vi "rad7.vi"() -> ()   [LabVIEW 2012]
uses:
  <vilib>/Platform/TimedLoop/XDataNode/timing_clust.ctl
  <vilib>/Platform/TimedLoop/XDataNode/nitl_modes.ctl
  <vilib>/Platform/TimedLoop/XDataNode/wakeup.ctl
  <vilib>/Instr/_visa.llb/VISA Configure Serial Port (Instr).vi
  <vilib>/Platform/TimedLoop/XDataNode/XDataNode.xnode
  <vilib>/Platform/TimedLoop/XDataNode/XDNodeRunTimeDep.lvlib
panel:
  out "String":string
  out "Numeric 2":i32
  in  "Path":path
  in  "VISA resource name":refnum<visa-resource-name>
  in  "Command":string
  out "Numeric":i32
  in  "Loop Time (s)":dbl
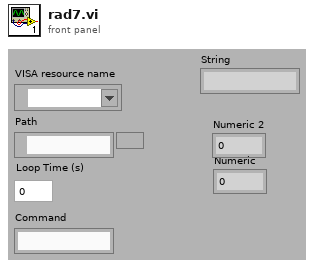
[diagram p1: front panel]
types:
  T1 = typedef "XDNodeRunTimeDep.lvlib/timing_clust.ctl" = cluster{"Expected End [f-1]":u64, "Actual End [f-1]":u64, "Finished Late? [f-1]":bool, "Expected End [i-1]":u64, "Actual End [i-1]":u64, "Finished Late? [i-1]":bool, "Expected Start [i]":u64, "Actual Start [i]":u64, "Expected Start [f]":u64, "Actual Start [f]":u64, "Source Name":string, "Structure Name":string, "Period":i64, "Deadline":i64, "Offset":i64, "Start":i64, "Priority":i32, "Timeout":i32, "Mode":T2, "Wakeup Reason":T3, "Error":errorcluster, "Source Type":string, "Secondary Source Type":string, "Global End Time":u64, "Global Start Time":u64, "Frame Duration":u64, "Iteration Duration":u64, "Assigned CPU":i32, "I/O Scan Engine Mode":u32}
  T2 = typedef "XDNodeRunTimeDep.lvlib/nitl_modes.ctl" = enum32{"No Change", "Process missed periods, maintain original phase", "Discard missed periods, maintain original phase", "Process missed periods, ignore original phase", "Discard missed periods, ignore original phase"}
  T3 = typedef "XDNodeRunTimeDep.lvlib/wakeup.ctl" = enum32{"Normal", "Aborted", "Asynchronous wakeup", "Timing source error", "Timed loop error", "Timeout"}
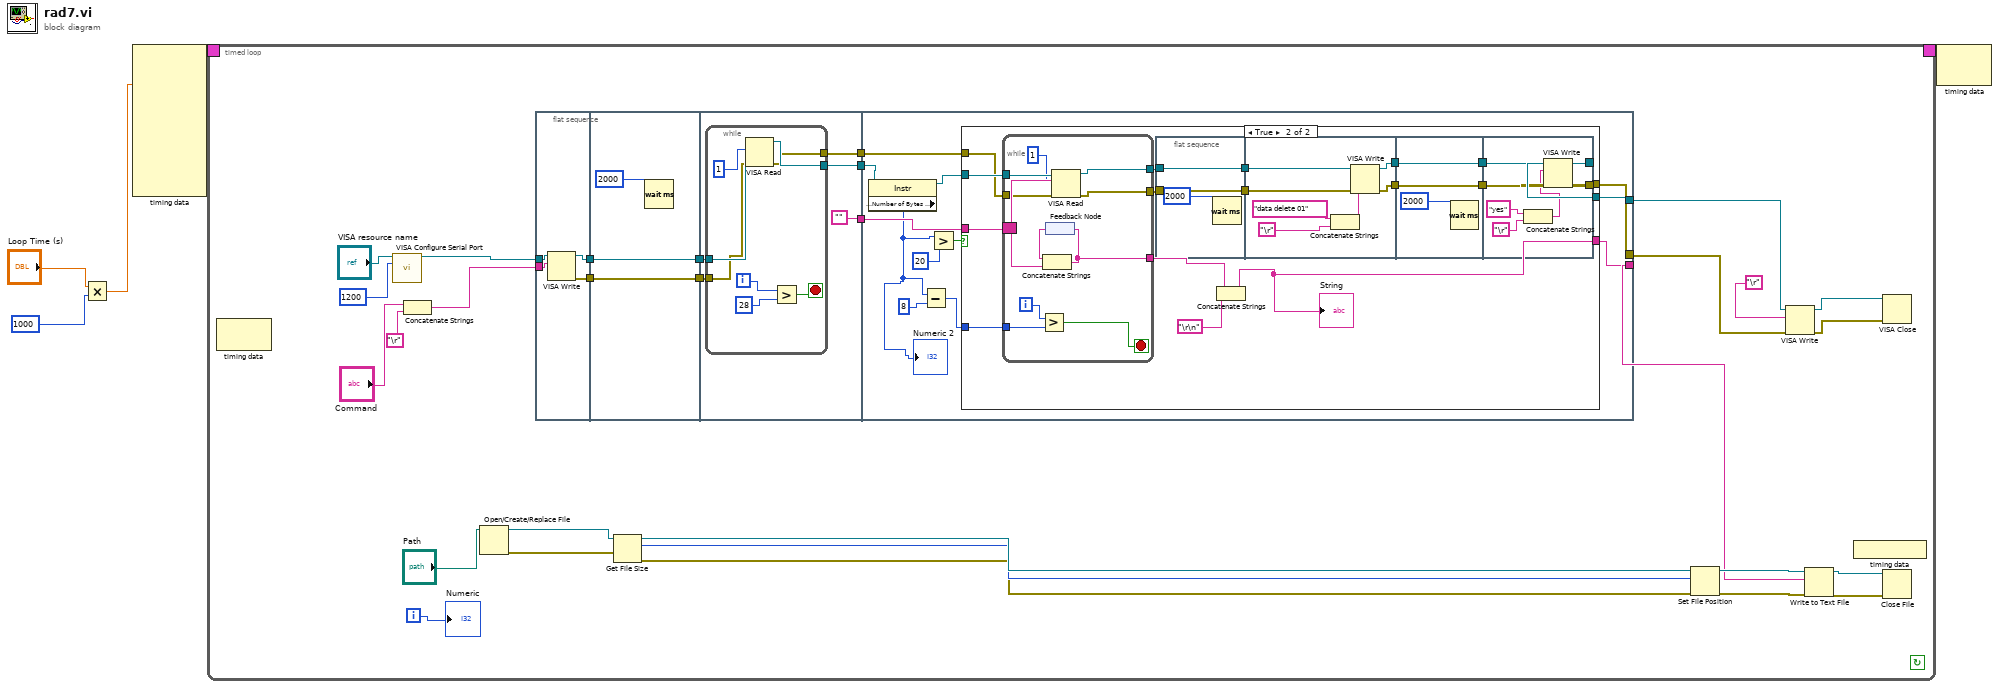
[diagram p0: block diagram]
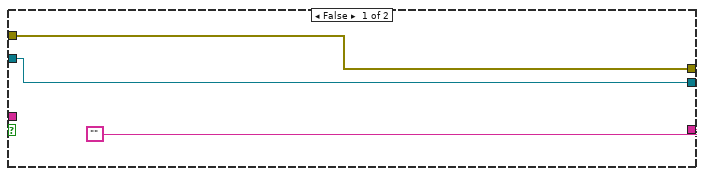
[diagram p2: hidden frame]
diagram:
  n1 = Multiply(x="Loop Time (s)", y=1000) -> (x*y=w1:dbl)
  n2 = node-c288(w1) -> (w5:T1)  [unwired: 8 in]
  n3 = timed-loop {
    timing: w5 -> [_]
    timing-out: [_] -> w4
    i -> [w30]
    stop <- _ continue-if-true
    n4 = node-c288() -> ()  [unwired: 1 in, 1 out]
    n5 = call-poly "VISA Configure Serial Port"("VISA resource name"="VISA resource name", "baud rate (9600)"=1200) -> ("VISA resource name out"=w16:refnum<visa-resource-name>)  [unwired: 12 in, 1 out]
    n6 = Concatenate Strings("Command", "\r") -> (w15:string)
    n7 = Open/Create/Replace File(file path (use dialog)="Path") -> (refnum out=w34:refnum<file>, error out=w33:errorcluster)  [unwired: 5 in, 1 out]
    n8 = flat-sequence {
      tunnel: w15 -> [w39]
      tunnel: w16 -> [w38]
      tunnel: [w37] -> w11
      tunnel: [w36] -> w9
      tunnel: w11 -> [w42]
      tunnel: [w42] -> w10
      tunnel: w9 -> [w41]
      tunnel: [w41] -> w8
      tunnel: [w47] -> w19
      tunnel: [""] -> w18
      tunnel: [w45] -> w17
      tunnel: w10 -> [w44]
      tunnel: w8 -> [w43]
      tunnel: [w67] -> w12
      tunnel: w19 -> [w65]
      tunnel: w18 -> [w66]
      tunnel: [w59] -> w13
      tunnel: w17 -> [w61]
      tunnel: [w60] -> w14
      frame #0 {
        n9 = VISA Write(VISA resource name=w38, write buffer=w39) -> (VISA resource name out=w37:refnum<visa-resource-name>, error out=w36:errorcluster)  [unwired: 1 in, 1 out]
      }
      frame #1 {
        n10 = Wait (ms)(milliseconds to wait=2000) -> ()  [unwired: 1 out]
      }
      frame #2 {
        n11 = while {
          tunnel: w44 -> [w54]
          tunnel: [w50] -> w47
          tunnel: w43 -> [w49]
          tunnel: [w48] -> w45
          i -> [w53]
          stop <- w51 stop-if-true
          n12 = VISA Read(VISA resource name=w54, byte count=1, error in (no error)=w49) -> (VISA resource name out=w50:refnum<visa-resource-name>, error out=w48:errorcluster)  [unwired: 2 out]
          n13 = Greater?(x=w53, y=28) -> (0:w51:bool)
        }
      }
      frame #3 {
        n14 = property class="Instr"(reference=w65) -> (reference out=w64:refnum<visa-resource-name>, "Serial Settings:Number of Bytes at Serial Port"=w57:u32)  [unwired: 1 in, 1 out]
        "Numeric 2" <- w57
        n15 = Subtract(x=w57, y=8) -> (x-y=w56:u32)
        n16 = Greater?(x=w57, y=20) -> (0:w63:bool)
        n17 = case shown="True" w63 {
          tunnel: [w70 w81] -> w67
          tunnel: w66 -> [_ w87]
          tunnel: ["" w73] -> w59
          tunnel: w64 -> [w70 w86]
          tunnel: w56 -> [_ w85]
          tunnel: w61 -> [w69 w80]
          tunnel: [w69 w78] -> w60
          frame False {
          }
          frame True {
            n18 = while {
              tunnel: w86 -> [w114]
              border: w87 -> [_]
              tunnel: [w115] -> w83
              tunnel: w85 -> [w112]
              tunnel: [w110] -> w82
              tunnel: w80 -> [w109]
              tunnel: [w108] -> w79
              i -> [w116]
              stop <- w111 stop-if-true
              n19 = Greater?(x=w116, y=w112) -> (0:w111:bool)
              n20 = feedback #1() -> (w117:string)
              n21 = VISA Read(VISA resource name=w114, byte count=1, error in (no error)=w109) -> (VISA resource name out=w110:refnum<visa-resource-name>, read buffer=w118:string, error out=w108:errorcluster)  [unwired: 1 out]
              n22 = Concatenate Strings(w117, w118) -> (w115:string)
              n23 = feedback-in #1(w115) -> ()
            }
            n24 = flat-sequence {
              tunnel: w79 -> [w89]
              tunnel: w82 -> [w90]
              tunnel: [w90] -> w72
              tunnel: [w89] -> w71
              tunnel: [w94] -> w77
              tunnel: [w91] -> w75
              tunnel: w72 -> [w93]
              tunnel: w71 -> [w92]
              tunnel: w77 -> [w100]
              tunnel: [w100] -> w76
              tunnel: w75 -> [w99]
              tunnel: [w99] -> w74
              tunnel: w76 -> [w104]
              tunnel: [w103] -> w81
              tunnel: w74 -> [w102]
              tunnel: [w101] -> w78
              frame #0 {
                n25 = Wait (ms)(milliseconds to wait=2000) -> ()  [unwired: 1 out]
              }
              frame #1 {
                n26 = Concatenate Strings("data delete 01", "\r") -> (w95:string)
                n27 = VISA Write(VISA resource name=w93, write buffer=w95, error in (no error)=w92) -> (VISA resource name out=w94:refnum<visa-resource-name>, error out=w91:errorcluster)  [unwired: 1 out]
              }
              frame #2 {
                n28 = Wait (ms)(milliseconds to wait=2000) -> ()  [unwired: 1 out]
              }
              frame #3 {
                n29 = Concatenate Strings("yes", "\r") -> (w105:string)
                n30 = VISA Write(VISA resource name=w104, write buffer=w105, error in (no error)=w102) -> (VISA resource name out=w103:refnum<visa-resource-name>, error out=w101:errorcluster)  [unwired: 1 out]
              }
            }
            n31 = Concatenate Strings(w83, "\r\n") -> (w73:string)
            "String" <- w73
          }
        }
      }
    }
    n32 = Get File Size(file=w34, error in=w33) -> (refnum out=w25:refnum<file>, size (in bytes)=w23:i64, 0:w22:errorcluster)
    n33 = Set File Position(offset (in bytes) (0)=w23, refnum=w25, error in=w22) -> (refnum out=w24:refnum<file>, error out=w21:errorcluster)  [unwired: 1 in]
    n34 = VISA Write(VISA resource name=w12, write buffer="\r", error in (no error)=w14) -> (VISA resource name out=w7:refnum<visa-resource-name>, error out=w6:errorcluster)  [unwired: 1 out]
    n35 = Write to Text File(file (use dialog)=w24, text=w13, error in=w21) -> (refnum out=w32:refnum<file>, error out=w31:errorcluster)  [unwired: 1 in, 1 out]
    n36 = node-c288() -> ()  [unwired: 1 out]
    n37 = VISA Close(VISA resource name=w7, error in (no error)=w6) -> ()  [unwired: 1 out]
    n38 = Close File(refnum=w32, error in=w31) -> ()  [unwired: 2 out]
    "Numeric" <- w30
  }
  n39 = node-c288(w4) -> ()  [unwired: 1 out]
